vi "Load Config File.vi"(11 "File Path":path) -> (1 "value":T1={"Client-ID"="MQTTCLIENT-001", "Server Address"="localhost", "Server Port"=1883})   [LabVIEW 2024, in "MQTTClient.lvlib"]
doc: "<b>Note:</b> This VI was modified by the <b>Validate DQMH Module</b> tool to turn off automatic error handling."
uses:
  MQTTClient.lvlib
  Config--cluster.ctl
  <userlib>/_OpenG.lib/file/file.llb/File Exists - Scalar__ogtk.vi
  <vilib>/Utility/xml.llb/Read From XML File(string).vi
  <userlib>/_OpenG.lib/file/file.llb/openg_file.lvlib
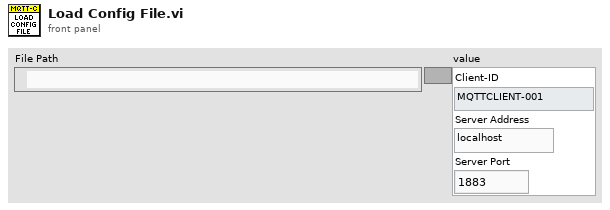
[diagram p1: front panel]
types:
  T1 = typedef "MQTTClient.lvlib/Config--cluster.ctl" = cluster{"Client-ID":string, "Server Address":string, "Server Port":u16}
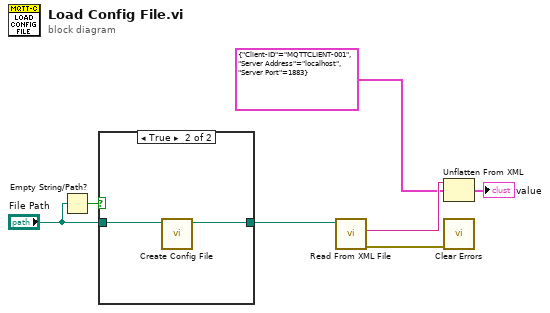
[diagram p0: block diagram]
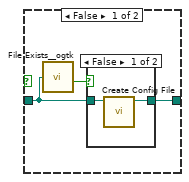
[diagram p2: hidden frame]
diagram:
  n1 = Empty String/Path?(string/path="File Path") -> (empty?=w3:bool)
  n2 = case shown="True" w3 {
    tunnel: [w10 w14] -> w6
    tunnel: "File Path" -> [w9 w15]
    frame False {
      n3 = call-poly <userlib>:"File Exists__ogtk.vi"("file path"=w9) -> ("exists"=w8:bool)  [unwired: 6 in, 1 out]
      n4 = case shown="False" w8 {
        tunnel: w9 -> [w12 w13]
        tunnel: [w11 w13] -> w10
        frame False {
          n5 = call "Create Config File.vi"("XML File Path"=w12) -> ("XML File Path(duplicate)"=w11:path)  [unwired: 10 in]
        }
        frame True {
        }
      }
    }
    frame True {
      n6 = call "Create Config File.vi"("XML File Path"=w15) -> ("XML File Path(duplicate)"=w14:path)  [unwired: 10 in]
    }
  }
  n7 = call-poly <vilib>:"Read From XML File.vi"("XML File Path"=w6) -> ("error out"=w5:errorcluster, "XML Elements"=w7:string)  [unwired: 8 in, 1 out]
  n8 = Unflatten From XML(xml string=w7, type=T1 {"Client-ID"="MQTTCLIENT-001", "Server Address"="localhost", "Server Port"=1883} ("Configuration")) -> (value=→"value":T1)  [unwired: 1 in, 1 out]
  n9 = call <vilib>:"Clear Errors.vi"("error in (no error)"=w5) -> ()  [unwired: 5 in, 2 out]
